vi "DPCODot1400.vi"() -> ()   [LabVIEW 2011]
uses:
  <vilib>/vision/Image Controls.llb/IMAQ Image.ctl
  <vilib>/Utility/importsl/GetValueByPointer/datatype.ctl
  <vilib>/Utility/importsl/GetValueByPointer/GetValueByPointer.xnode
  National Instruments/LabVIEW 2011/resource/lvimptsl.dll
panel:
  in  "Handle":u64 caption="Handle (0 for new)- stored default has to be 0!"
  out "binning":i32=1
  out "save all?":bool
  out "image":i32
  out "run":i32
  out "error":errorcluster
  # "no binning\nnew: localPointer\nsmall delay~300ms"
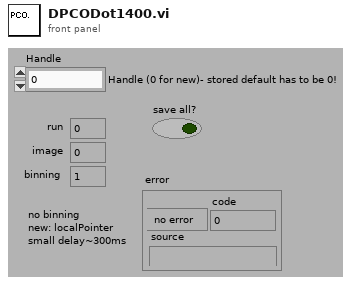
[diagram p1: front panel]
types:
  T1 = enum16{"None/#Datasets", "Clear", "TagValueOf#", "AddValues", "ReadValue", "ChangeValue", "Get all"}
  T2 = typedef "IMAQ Image.ctl" = refnum<image>
  T3 = cluster{"Center":cluster{dbl, dbl}, "Rotate (rad)":dbl, "MirrorY":bool, "Scale":dbl}
  T4 = enum16{"status", "createIMAQ", "getIMAQ", "getNumber", "deleteIMAQ", "deleteAll", "MemoryUsage", "GetAccess", "DecreaseAccess", "ActualIndex", "ElementToNumber"}
  T5 = enum16{"status", "saveMeta", "getMeta", "deleteMeta", "deleteAll", "MemoryUsage"}
  T6 = enum16{"status", "createIMAQ", "getIMAQ", "getNumber", "deleteIMAQ", "deleteAll", "MemoryUsage", "GetAccess", "DecreaseAccess", "ActualIndex"}
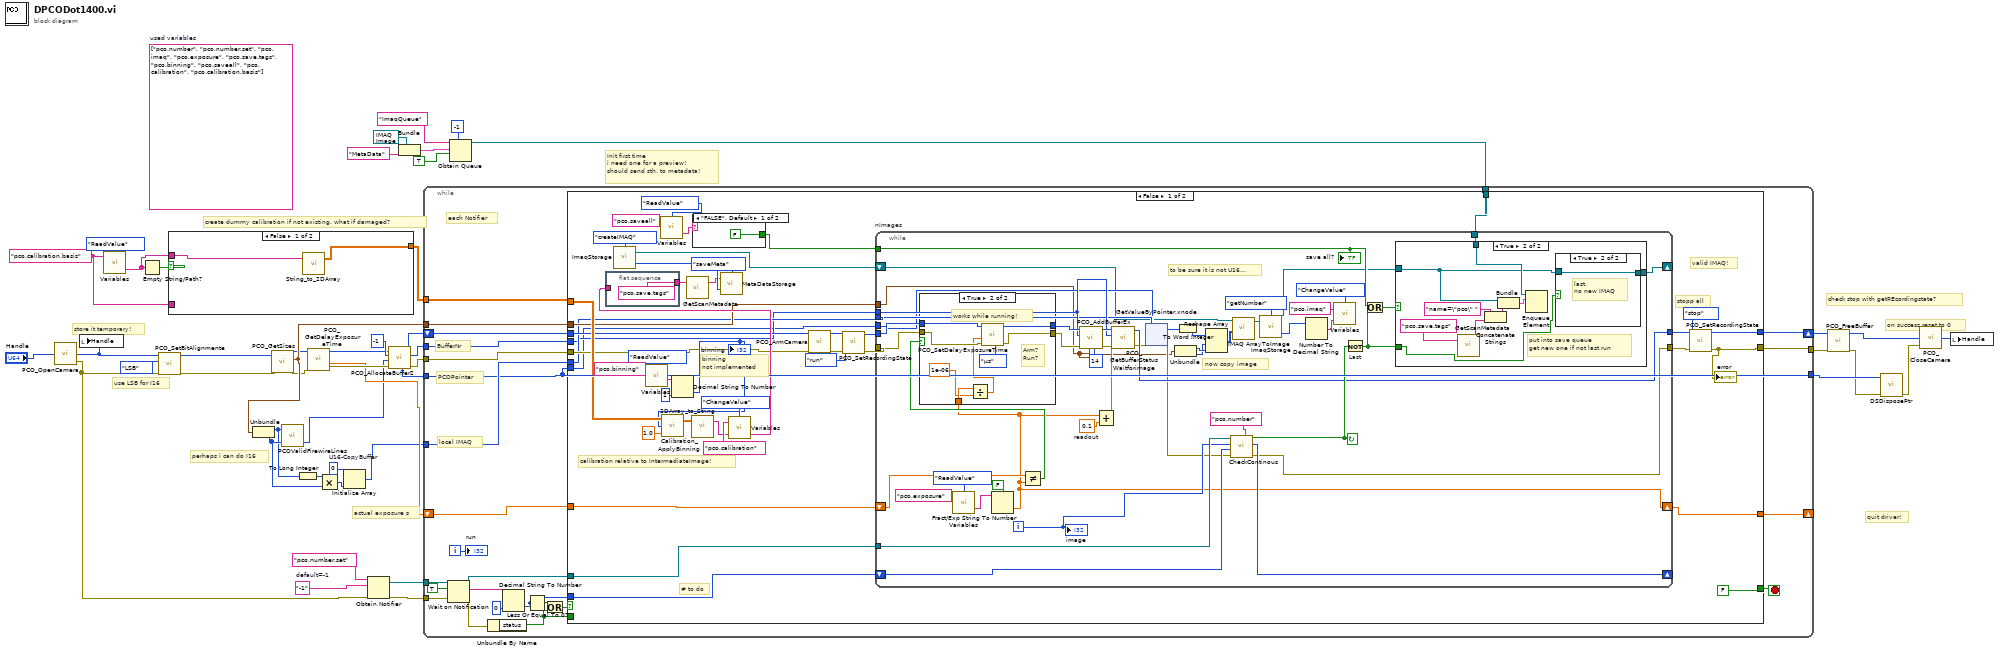
[diagram p0: block diagram]
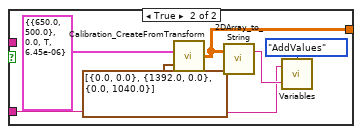
[diagram p2: hidden frame]
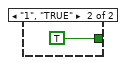
[diagram p3: hidden frame]
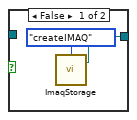
[diagram p6: hidden frame]
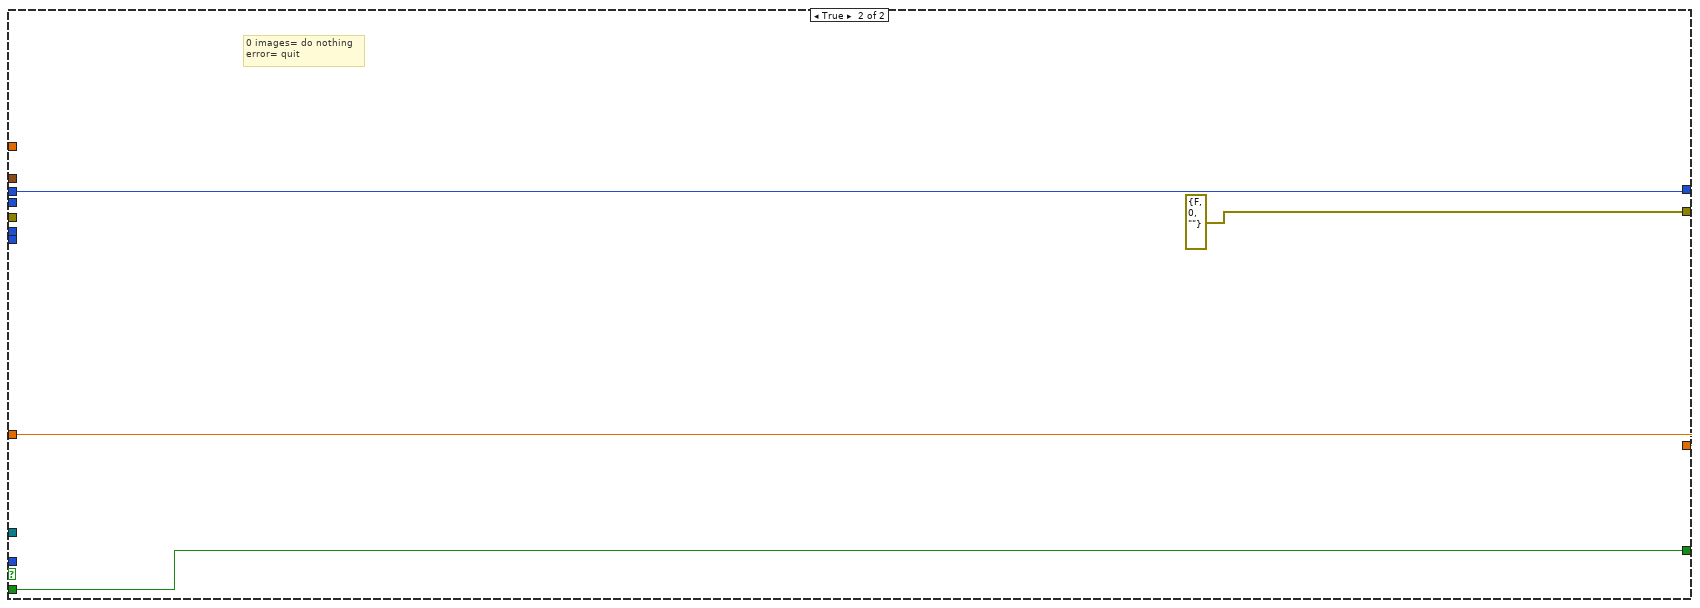
[diagram p7: hidden frame]
diagram:
  w8 = i16 0  # U16-CopyBuffer
  w33 = "pco.calibration.basis" ("Tag in")
  (unwired) string[] ["pco.number", "pco.number.set", "pco.imaq", "pco.exposure", "pco.save.tags", "pco.binning", "pco.saveall", "pco.calibration", "pco.calibration.basis"]  # used variables
  w38 = "-1"  # default=-1
  # "perhaps i can do I16"
  # "check stop with getREcordingstate?"
  # "Init first time\ni need one for a preview!\nshould send sth. to metadata!"
  # "on success reset to 0"
  # "store it temporary!"
  # "use LSB for I16"
  # "create dummy calibration if not existing. what if damaged?"
  # "actual exposure s"
  # "quit driver!"
  n1 = call "PCO_OpenCamera.vi"("Handle (0 for new)"="Handle") -> ("error out"=w30:errorcluster, "Handle Out"=w28:u64)  [unwired: 1 in, 2 out]
  n2 = local write "Handle"(w28) -> ()
  n3 = call "Variables.vi"("Tag in"=w33, "Command"=T1."ReadValue") -> ("value out"=w32:string)  [unwired: 1 in, 2 out]
  n4 = Empty String/Path?(string/path=w32) -> (empty?=w35:bool)
  n5 = call "PCO_SetBitAlignmente.vi"("error in (no error)"=w30, "wBitAlignment"=enum16{"MSB", "LSB"}."LSB", "Handle"=w28) -> ("error out"=w2:errorcluster, "Handle Out"=w1:u64)  [unwired: 7 out]
  n6 = case shown="False" w35 {
    tunnel: w32 -> [w48 _]
    tunnel: [w49 w55] -> w34
    tunnel: w33 -> [_ w52]
    frame False {
      n7 = call "String_to_2DArray.vi"("String"=w48) -> ("Array"=w49:dbl[][])  [unwired: 3 in, 1 out]
    }
    frame True {
      n8 = call "Calibration_CreateFromTransform.vi"("sample points"=cluster{dbl, dbl}[] [{0.0, 0.0}, {1392.0, 0.0}, {0.0, 1040.0}], "Transform (Center first)"=T3 {"Center"={650.0, 500.0}, "Rotate (rad)"=0.0, "MirrorY"=TRUE, "Scale"=6.45e-06}) -> ("CalibrationCoordinates: x,x',y,y'..."=w55:dbl[][])
      n9 = call "2DArray_to_String.vi"("Array"=w55) -> ("String 1"=w53:string)  [unwired: 3 in, 1 out]
      n10 = call "Variables.vi"("value"=w53, "Tag in"=w52, "Command"=T1."AddValues") -> ()  [unwired: 3 out]
    }
  }
  n11 = call "PCO_GetSizes.vi"("error in (no error)"=w2, "Handle"=w1) -> ("error out"=w15:errorcluster, "ActRes"=w26:cluster{"wXResAct":u16, "wYResAct":u16}, "Handle Out"=w22:u64)  [unwired: 7 out]
  n12 = Unbundle(w26) -> ("wXResAct"=w11:u16, "wYResAct"=w12:u16)
  n13 = call "PCOValidFirewireLines.vi"("wYResAct"=w12, "wXResAct"=w11) -> ("ValidBytes"=w13:u32)  [unwired: 1 out]
  n14 = To Long Integer(number=w11) -> (32bit integer=w10:i32)
  n15 = call "PCO_GetDelayExposureTime.vi"("error in (no error)"=w15, "Handle"=w22) -> ("error out"=w24:errorcluster, "Exposure [s]"=w14:dbl, "Handle Out"=w21:u64)  [unwired: 7 out]
  n16 = Multiply(x=w10, y=w12) -> (x*y=w9:i32)
  n17 = Initialize Array(w8, w9) -> (w7:i16[])
  n18 = Obtain Notifier(name (unnamed)="pco.number.set", notification data type=w38, error in (no error)=w30) -> (notifier out=w46:refnum<notifier>, error out=w37:errorcluster)  [unwired: 1 in, 1 out]
  n19 = call "PCO_AllocateBuffer2.vi"("error in (no error)"=w24, "PointerSize (bytes)"=w13, "sBufNr"=i16 -1, "Handle"=w21) -> ("error out"=w23:errorcluster, "sBufNr out"=w19:i16, "Handle Out"=w20:u64, "BufferPointer"=w6:u64)  [unwired: 2 in, 2 out]
  n20 = Bundle("New Image"=T2 refnum, "MetaData") -> (w41:cluster{"New Image":T2, string})  [unwired: 1 out]
  n21 = Obtain Queue(max queue size (-1, unlimited)=-1, name (unnamed)="ImaqQueue", element data type=w41, create if not found? (T)=TRUE) -> (queue out=w39:refnum<queue>)  [unwired: 1 in, 2 out]
  n22 = while {
    shift-right: [w67] -> _
    shift-left: w14 -> [w68]
    tunnel: w46 -> [w78]
    tunnel: w39 -> [w77]
    tunnel: [w79] -> w18
    tunnel: w23 -> [w65]
    tunnel: w37 -> [w64]
    shift-right: [w62] -> w17
    shift-left: w20 -> [w63]
    tunnel: w34 -> [w60]
    tunnel: w26 -> [w59]
    tunnel: w7 -> [w57]
    tunnel: w6 -> [w56]
    tunnel: w19 -> [w58]
    tunnel: [w56] -> w5
    i -> [w74]
    stop <- w80 stop-if-true
    # "BufferNr"
    # "PCOPointer"
    # "local IMAQ"
    # "each Notifier"
    n23 = Wait on Notification(notifier=w78, ignore previous (F)=TRUE, error in (no error)=w64) -> (notifier out=w76:refnum<notifier>, notification=w66:string, error out=w73:errorcluster)  [unwired: 2 out]
    n24 = Unbundle By Name(w73) -> ("status"=w69:bool)
    n25 = Decimal String To Number(string=w66, default (0L)=0 ("default (0 I32)")) -> (number=w72:i32)  [unwired: 2 out]
    n26 = Less Or Equal To 0?(x=w72) -> (x <= 0?=w71:bool)
    n27 = Or(x=w71, y=w69) -> (x .or. y?=w70:bool)
    n28 = case shown="False" w70 {
      tunnel: [FALSE ("status") w213] -> w80
      tunnel: [w84 errorcluster {"status"=FALSE, "code"=0, "source"=""} ("error out")] -> w79
      tunnel: w77 -> [w124 _]
      tunnel: w76 -> [w123 _]
      tunnel: w72 -> [w121 _]
      tunnel: w69 -> [_ w213]
      tunnel: w68 -> [w120 w211]
      tunnel: [w107 w211] -> w67
      tunnel: w65 -> [w87 _]
      tunnel: w63 -> [w86 w210]
      tunnel: [w85 w210] -> w62
      tunnel: w60 -> [w102 _]
      tunnel: w59 -> [w93 _]
      tunnel: w57 -> [w83 _]
      tunnel: w58 -> [w82 _]
      tunnel: w56 -> [w81 _]
      frame False {
        # "binning\nnot implemented"
        # "calibration relative to IntermediateImage!"
        # "valid IMAQ!"
        # "# to do"
        # "stopp all"
        n29 = flat-sequence {
          tunnel: ["pco.save.tags" ("Tag (save.tags)")] -> w113
          tunnel: w103 -> [_]
          frame #0 {
          }
        }
        n30 = call "ImaqStorage.vi"("Command"=T4."createIMAQ") -> ("Number out"=w115:i32, "IMAQ out"=w97:T2)  [unwired: 2 in]
        n31 = call "Variables.vi"("Tag in"="pco.binning", "Command"=T1."ReadValue") -> ("value out"=w118:string)  [unwired: 1 in, 2 out]
        n32 = call "Variables.vi"("Tag in"="pco.saveall", "Command"=T1."ReadValue") -> ("value out"=w110:string)  [unwired: 1 in, 2 out]
        n33 = Decimal String To Number(string=w118, default (0L)=1 ("Standard (0 I32)")) -> (number=w98:i32)  [unwired: 2 out]
        "binning" <- w98
        n34 = call "Calibration_ApplyBinning.vi"("magnification"=1.0, "Binning"=w98, "CalibrationCoordinates: x,x',y,y'..."=w102) -> ("CalibrationCoordinates: x,x',y,y'... 2"=w100:dbl[][])  [unwired: 1 out]
        n35 = call "GetScanMetadata.vi"("Tag (save.tags)"=w113) -> ("Metadata"=w114:string)  [unwired: 1 in, 1 out]
        n36 = call "2DArray_to_String.vi"("Array"=w100) -> ("String 1"=w101:string)  [unwired: 3 in, 1 out]
        n37 = case shown="\"FALSE\", Default" w110 {
          tunnel: [FALSE TRUE] -> w109
          frame "FALSE", Default {
          }
          frame "1", "TRUE" {
          }
        }
        n38 = call "MetaDataStorage.vi"("Number"=w115, "Meta in"=w114, "Command"=T5."saveMeta") -> ()  [unwired: 2 out]
        n39 = call "Variables.vi"("value"=w101, "Tag in"="pco.calibration", "Command"=T1."ChangeValue") -> ("value out"=w103:string)  [unwired: 2 out]
        n40 = call "PCO_ArmCamera.vi"("error in (no error)"=w87, "Handle"=w86) -> ("error out"=w91:errorcluster, "Handle Out"=w92:u64)  [unwired: 8 out]
        n41 = call "PCO_SetRecordingState.vi"("error in (no error)"=w91, "wRecState"=enum16{"stop", "run"}."run", "Handle"=w92) -> ("error out"=w90:errorcluster, "Handle Out"=w89:u64)  [unwired: 7 out]
        n42 = while "nImages" {
          tunnel: w124 -> [w175]
          tunnel: w123 -> [w163]
          shift-right: [w161] -> _
          shift-left: w121 -> [w157]
          tunnel: [w152] -> w94
          shift-right: [w174] -> _
          shift-left: w97 -> [w136]
          tunnel: w109 -> [w158]
          tunnel: w89 -> [w155]
          tunnel: [w144] -> w95
          shift-right: [w145] -> w107
          shift-left: w120 -> [w165]
          tunnel: w90 -> [w154]
          tunnel: w93 -> [w131]
          tunnel: w83 -> [w138]
          tunnel: w82 -> [w143]
          tunnel: w81 -> [w137]
          i -> [w153]
          stop <- w162 continue-if-true
          w141 = 0.1  # readout
          # "now copy image"
          # "to be sure it is not U16..."
          n43 = call "Variables.vi"("Tag in"="pco.exposure", "Command"=T1."ReadValue") -> ("value out"=w168:string)  [unwired: 1 in, 2 out]
          n44 = Fract/Exp String To Number(use system decimal point (T)=FALSE, string=w168) -> (number=w145:dbl)  [unwired: 3 out]
          n45 = Not Equal?(x=w165, y=w145) -> (x != y?=w156:bool)
          n46 = case shown="True" w156 {
            tunnel: w155 -> [w188 w195]
            tunnel: w145 -> [_ w196]
            tunnel: [w188 w194] -> w148
            tunnel: w154 -> [w187 w192]
            tunnel: [w187 w193] -> w149
            frame False {
              # "same exposure"
            }
            frame True {
              # "Arm?\nRun?"
              # "works while running!"
              n47 = Divide(x=w196, y=1e-06) -> (x/y=w189:dbl)
              n48 = call "PCO_SetDelayExposureTime.vi"("wTimebaseExposure"=enum16{"ns", "µs", "ms"}."µs", "error in (no error)"=w192, "dwExposure"=w189, "Handle"=w195) -> ("error out"=w193:errorcluster, "Handle Out"=w194:u64)  [unwired: 2 in, 4 out]
            }
          }
          n49 = call "PCO_AddBufferEx.vi"("BitPerPixel"=u16 14, "Resolution"=w131, "error in (no error)"=w149, "sBufNr"=w143, "Handle"=w148) -> ("error out"=w147:errorcluster, "Handle Out"=w146:u64)  [unwired: 1 in, 4 out]
          n50 = Add(x=w145, y=w141) -> (x+y=w142:dbl)
          n51 = call "PCO_GetBufferStatusWaitforimage.vi"("error in"=w147, "expected seconds"=w142, "sBufNr"=w143, "Handle"=w146) -> ("error out"=w140:errorcluster, "Handle Out"=w144:u64)  [unwired: 1 out]
          n52 = xnode "GetValueByPointer.xnode"("Pointer"=w137, "InputType"=w138, "ErrorIn"=w140) -> ("Output"=w128:i16[], "ErrorOut"=w139:errorcluster)  [unwired: 1 in]
          n53 = Unbundle(w131) -> ("wXResAct"=w130:u16, "wYResAct"=w129:u16)
          n54 = To Word Integer(number=w128) -> (16bit integer=w132:i16[])
          n55 = Reshape Array(w132, w129, w130) -> (w133:i16[][])
          n56 = call "CheckContinous.vi"("notifier (var.Name / data)"=w163, "Numbers done"=w153, "Numbers to do"=w157, "error in (no error)"=w139, "Tag in (scan.number)"="pco.number" ("Tag in")) -> ("continue?"=w162:bool, "Numbers to do out"=w161:i32, "error out"=w152:errorcluster)  [unwired: 1 out]
          n57 = call "IMAQ ArrayToImage"("Image Pixels (I16)"=w133, "Image"=w136) -> ("Image Out"=w135:T2)  [unwired: 8 in, 1 out]
          n58 = call "ImaqStorage.vi"("IMAQ in"=w135, "Command"=T4."getNumber") -> ("Number out"=w159:i32, "IMAQ out"=w134:T2)  [unwired: 1 in]
          n59 = Number To Decimal String(number=w159) -> (decimal integer string=w172:string)  [unwired: 1 out]
          n60 = call "Variables.vi"("value"=w172, "Tag in"="pco.imaq", "Command"=T1."ChangeValue") -> ()  [unwired: 3 out]
          n61 = Not "Last"(x=w162) -> (.not. x?=w160:bool)
          n62 = Or(x=w158, y=w160) -> (x .or. y?=w173:bool)
          n63 = case shown="True" w173 {
            tunnel: w175 -> [_ w206]
            tunnel: w134 -> [w197 w200]
            tunnel: [w197 w201] -> w174
            tunnel: w160 -> [_ w198]
            frame False {
              # "last or all?"
              # "keep the IMAQ"
            }
            frame True {
              # "put into save queue\nget new one if not last run"
              n64 = call "GetScanMetadata.vi"("Tag (save.tags)"="pco.save.tags") -> ("Metadata"=w202:string)  [unwired: 1 in, 1 out]
              n65 = Concatenate Strings("name=\"pco\" " ("string"), w202) -> (w204:string)
              n66 = Bundle("IMAQ out"=w200, w204) -> (w203:cluster{"IMAQ out":T2, string})  [unwired: 1 out]
              n67 = Enqueue Element(queue=w206, element=w203) -> ()  [unwired: 1 in, 4 out]
              n68 = case shown="True" w198 {
                tunnel: [w207 w209] -> w201
                tunnel: w200 -> [_ w209]
                frame False {
                  n69 = call "ImaqStorage.vi"("Command"=T6."createIMAQ") -> ("IMAQ out"=w207:T2)  [unwired: 2 in, 1 out]
                }
                frame True {
                  # "last,\nno new IMAQ"
                }
              }
            }
          }
          "image" <- w153
          "save all?" <- w158
        }
        n70 = call "PCO_SetRecordingState.vi"("error in (no error)"=w94, "wRecState"=enum16{"stop", "run"}."stop", "Handle"=w95) -> ("error out"=w84:errorcluster, "Handle Out"=w85:u64)  [unwired: 7 out]
        "error" <- w84
      }
      frame True {
        # "0 images= do nothing\nerror= quit"
      }
    }
    "run" <- w74
  }
  n71 = call "PCO_FreeBuffer.vi"("error in (no error)"=w18, "Handle"=w17) -> ("error out"=w4:errorcluster, "Handle Out"=w16:u64)  [unwired: 1 in, 7 out]
  n72 = call <vilib>:"DSDisposePtr.vi"("error in (no error)"=w4, "Pointer"=w5) -> ("error out"=w3:errorcluster)  [unwired: 9 in]
  n73 = call "PCO_CloseCamera.vi"("error in (no error)"=w3, "Handle"=w16) -> ("Handle Out (success:0, otherwise input)"=w27:u32)  [unwired: 3 out]
  n74 = local write "Handle"(w27) -> ()
